vi "Start Measurement.vi"(8 "error in":errorcluster, 9 "pin map context":T3, 10 "measurement configuration":T1, 11 "gRPCid in":T2) -> (0 "error out":errorcluster, 2 "call id":T2, 3 "gRPCid out":T2)   [LabVIEW 2021, in "Measurement Client Template.lvlib"]
uses:
  Measurement Client Template.lvlib
  <vilib>/gRPC/Generated APIs/ni/measurementlink/measurement/v2/Measurement Service Client V2/RPC Messages/ni_measurementlink_PinMapContext.ctl
  <vilib>/gRPC/LabVIEW gRPC Library/Shared/grpcId.ctl
  controls/Measurement Configuration.ctl
  <vilib>/gRPC/Generated APIs/ni/measurementlink/measurement/v2/Measurement Service Client V2/RPC Messages/ni_measurementlink_measurement_v2_MeasureRequest.ctl
  <vilib>/gRPC/Generated APIs/ni/measurementlink/measurement/v2/Measurement Service Client V2/RPC Messages/google_protobuf_Any.ctl
  7061fa50-9f43-4eb3-8fe8-31484f53e761.vi
  <vilib>/gRPC/LabVIEW gRPC Library/Server API/Translate Protobuf Error.vi
  <vilib>/AdvancedString/1D String Array to Delimited String.vi
  <vilib>/gRPC/LabVIEW gRPC Library/Server API/Server/Get Server DLL Path.vi
  <vilib>/gRPC/Generated APIs/ni/measurementlink/measurement/v2/Measurement Service Client V2/Measurement Service Client V2.lvlib
  <vilib>/gRPC/LabVIEW gRPC Library/grpc-lvsupport-release.lvlib
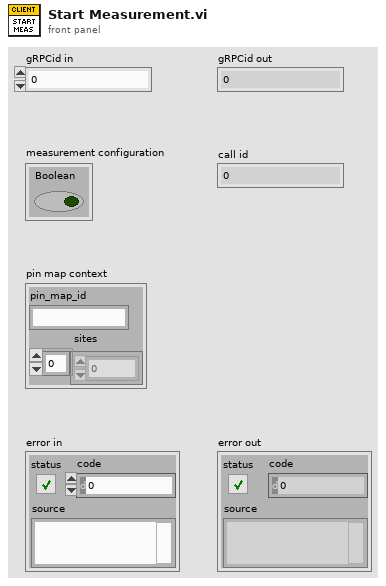
[diagram p1: front panel]
types:
  T1 = typedef "Measurement Client Template.lvlib/Measurement Configuration.ctl" = cluster{"Boolean":bool}
  T2 = typedef "grpc-lvsupport-release.lvlib/grpcId.ctl" = u64
  T3 = typedef "Measurement Service Client V2.lvlib/ni_measurementlink_PinMapContext.ctl" = cluster{"pin_map_id":string, "sites":i32[]}
  T4 = typedef "Measurement Service Client V2.lvlib/ni_measurementlink_measurement_v2_MeasureRequest.ctl" = cluster{"configuration_parameters":T5, "pin_map_context":T3}
  T5 = typedef "Measurement Service Client V2.lvlib/google_protobuf_Any.ctl" = cluster{"type_url":string, "value":u8[]}
  T6 = typedef "grpc-lvsupport-release.lvlib/Any.ctl" = cluster{"Type Url":string, "Bytes":u8[]}
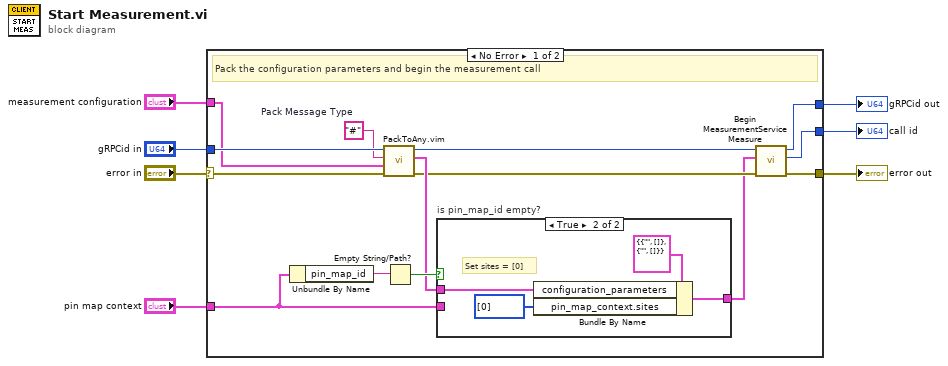
[diagram p0: block diagram]
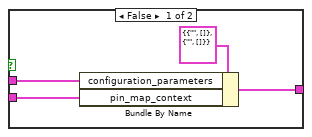
[diagram p2: hidden frame]
diagram:
  n1 = case shown="No Error" "error in" {
    selector: "error in" -> [w16 w30]
    tunnel: "pin map context" -> [w19 _]
    tunnel: "gRPCid in" -> [w17 _]
    tunnel: [w13 w30] -> w4
    tunnel: [w12 _] -> w3
    tunnel: [w11 _] -> w2
    tunnel: "measurement configuration" -> [w8 _]
    frame No Error {
      w9 = "#"  # Pack Message Type
      # "Pack the configuration parameters and begin the measurement call"
      n2 = Unbundle By Name(w19) -> ("pin_map_id"=w20:string)
      n3 = call "PackToAny.vim"("error in"=w16, "Data To Pack"=w8, "Message Type"=w9, "gRPCid in"=w17) -> ("error out"=w15:errorcluster, "Any"=w18:T6, "gRPCid out"=w10:u64)  [unwired: 5 in]
      n4 = Empty String/Path?(string/path=w20) -> (empty?=w21:bool)
      n5 = case "is pin_map_id empty?" shown="True" w21 {
        tunnel: [w25 w29] -> w14
        tunnel: w19 -> [w23 _]
        tunnel: w18 -> [w22 w28]
        frame False {
          n6 = Bundle By Name(cluster=T4 {"configuration_parameters"={"type_url"="", "value"=[]}, "pin_map_context"={"pin_map_id"="", "sites"=[]}} ("Request Data"), "configuration_parameters"=w22, "pin_map_context"=w23) -> (w25:T4)
        }
        frame True {
          # "Set sites = [0]"
          n7 = Bundle By Name(cluster=T4 {"configuration_parameters"={"type_url"="", "value"=[]}, "pin_map_context"={"pin_map_id"="", "sites"=[]}} ("Request Data"), "configuration_parameters"=w28, "pin_map_context.sites"=i32[] [0]) -> (w29:T4)
        }
      }
      n8 = call <vilib>:"Begin MeasurementService Measure.vi"("error in"=w15, "Request Data"=w14, "gRPC ID"=w10) -> ("error out"=w13:errorcluster, "Call Id Out"=w12:T2, "gRPC ID out"=w11:T2)  [unwired: 6 in]
    }
    frame Error {
      # "Pass"
    }
  }
  "error out" <- w4
  "call id" <- w3
  "gRPCid out" <- w2
